vi "Test_Copy_Raw_Memory_To_Image_Greyscale.vi"(8 "error in (no error)":errorcluster, 11 "Test Case In":refnum<class "Image.lvclass">) -> (0 "error out":errorcluster, 3 "Test Case Out":refnum<class "Image.lvclass">)   [LabVIEW 2020, in "g_ar_toolkit.test.lvlib" / "Image.lvclass"]
uses:
  Image.lvclass
  Image.lvclass/Image.ctl
  g_ar_toolkit.image/g_ar_toolkit.image.lvlib
  g_ar_toolkit.image/Raw Memory Information Dimension.ctl
  g_ar_toolkit.image/Raw Memory Information.ctl
  g_ar_toolkit.image/CreateEmptyImageGreyscale.vi
  g_ar_toolkit.image/Image Size (Fixed).ctl
  4993e8ee-a06a-463a-9684-69129f64d5ce.vi
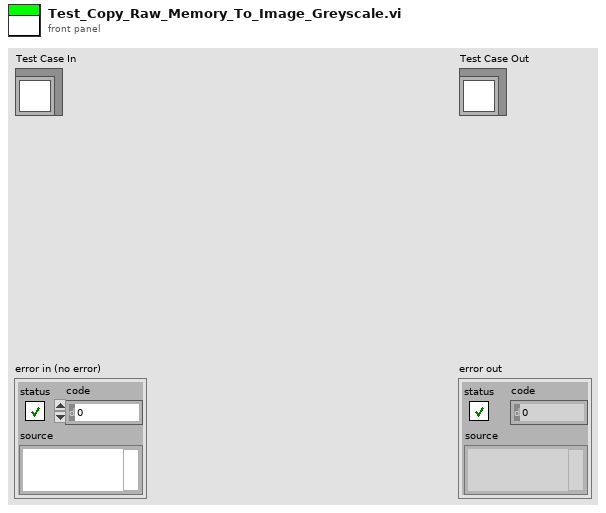
[diagram p1: front panel]
types:
  T1 = typedef "g_ar_toolkit.image.lvlib/Image Size (Fixed).ctl" = cluster{"Width":u16, "Height":u16}
  T2 = typedef "g_ar_toolkit.image.lvlib/Raw Memory Information.ctl" = cluster{"Memory Address":u64, "Dimension 0":T3, "Dimension 1":T3}
  T3 = typedef "g_ar_toolkit.image.lvlib/Raw Memory Information Dimension.ctl" = cluster{"Size":u16, "Stride":u32}
  T4 = cluster{"pointer":u64, "size_0":u32, "stride_0":i32, "size_1":u32, "stride_1":i32, "element size":u32, "subarray?":bool}
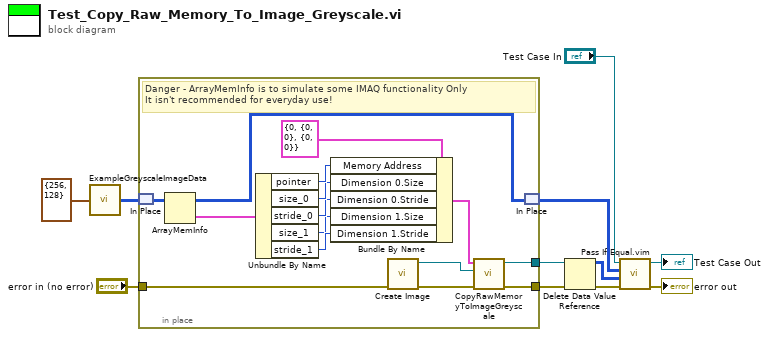
[diagram p0: block diagram]
diagram:
  n1 = call "ExampleGreyscaleImageData.vi"("Image Size"=T1 {"Width"=256, "Height"=128}) -> ("GreyscaleImage"=w2:u8[][])
  n2 = in-place {
    in-place-border: [w17] -> w8
    in-place-border: "error in (no error)" -> [w15]
    in-place-border: [w14] -> w5
    # "Danger - ArrayMemInfo is to simulate some IMAQ functionality Only\nIt isn't recommended for everyday use!"
    n3 = in-place-match #1(w2) -> (w13:u8[][])
    n4 = ArrayMemInfo(3:w13) -> (0:w26:T4, 1:w12:u8[][])
    n5 = Unbundle By Name(w26) -> ("pointer"=w25:u64, "size_0"=w23:u32, "stride_0"=w22:i32, "size_1"=w20:u32, "stride_1"=w21:i32)
    n6 = Bundle By Name(cluster=T2 {"Memory Address"=0, "Dimension 0"={"Size"=0, "Stride"=0}, "Dimension 1"={"Size"=0, "Stride"=0}} ("Source"), "Memory Address"=w25, "Dimension 0.Size"=w23, "Dimension 0.Stride"=w22, "Dimension 1.Size"=w20, "Dimension 1.Stride"=w21) -> (w18:T2)
    n7 = call-poly "Create Image.vi"("error in (no error)"=w15) -> ("error out"=w16:errorcluster, "New Greyscale Image"=w24:refnum<data-value>)  [unwired: 9 in]
    n8 = call "CopyRawMemoryToImageGreyscale.vi"("error in (no error)"=w16, "Greyscale Destination Image"=w24, "Source"=w18) -> ("error out"=w14:errorcluster, "Greyscale Destination Image (duplicate)"=w17:refnum<data-value>)  [unwired: 7 in]
    n9 = in-place-match #1(w12) -> (w3:u8[][])
  }
  n10 = Delete Data Value Reference(data value reference=w8, error in=w5) -> (data value=w7:u8[][], error out=w4:errorcluster)
  n11 = call "Pass If Equal.vim"("error in (no error)"=w4, "Actual"=w7, "Expected"=w3, "LUnit Test Case In"="Test Case In") -> ("error out"=→"error out":errorcluster, "LUnit Test Case Out"=→"Test Case Out":refnum<class "Image.lvclass">)  [unwired: 6 in]
